vi "ModifyOneRecordTo2DListCtrl.vi"(10 "arr data":string[](array[string]), 11 "multiple list in":refnum<vi>) -> (3 "multiple list out":refnum<vi>)   [LabVIEW 2018, in "Library-Ctrl.lvlib"]
uses:
  Library-Ctrl.lvlib
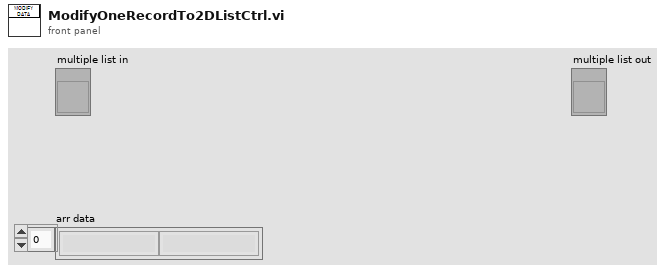
[diagram p1: front panel]
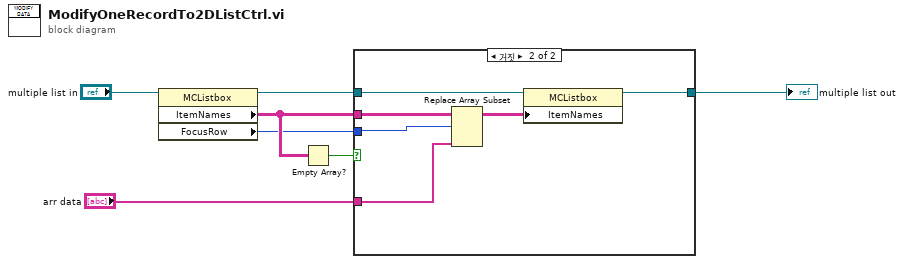
[diagram p0: block diagram]
diagram:
  n1 = property class="MCListbox"(reference="multiple list in") -> (reference out=w6:refnum<vi>, "ItemNames"=w3:string[][], "FocusRow"=w1:i32)  [unwired: 1 in, 1 out]
  n2 = Empty Array?(array=w3) -> (empty?=w2:bool)
  n3 = case shown="거짓" w2 {
    tunnel: w6 -> [w8 w14]
    tunnel: [w8 w12] -> w5
    tunnel: "arr data" -> [_ w11]
    tunnel: w3 -> [_ w10]
    tunnel: w1 -> [_ w9]
    frame True {
    }
    frame False {
      n4 = Replace Array Subset(array=w10, new element=w11, index (row)=w9) -> (w13:string[][])  [unwired: 1 in]
      n5 = property class="MCListbox"(reference=w14, "ItemNames"=w13) -> (reference out=w12:refnum<vi>)  [unwired: 1 in, 1 out]
    }
  }
  "multiple list out" <- w5
